vi "onDestroy.vi"(8 "error in (no error)":errorcluster, 11 "MeasuringDevice":refnum<class "MeasuringDevice.lvclass">) -> (0 "error out":errorcluster, 3 "MeasuringDevice out":refnum<class "MeasuringDevice.lvclass">)   [LabVIEW 2019, in "MeasuringDevice.lvclass"]
doc: "JKI State Machine Objects (SMO) 1.3.0.56\nJKI - JKI\nCopyright (c) 2017, JKI"
uses:
  MeasuringDevice.lvclass
  CircularBuffer/CircularBuffer.lvclass
  C:/Program Files (x86)/National Instruments/LabVIEW 2019/vi.lib/JKI/JKI SMO/SMO/SMO.lvclass
  Device/Device.lvclass
  <vilib>/JKI/JKI SMO/SMO/SMO.lvclass
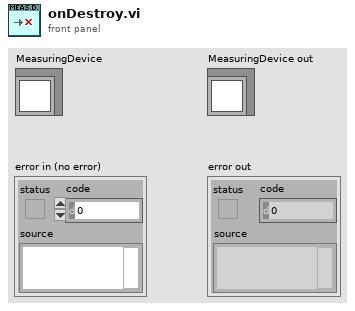
[diagram p1: front panel]
types:
  T1 = typedef "MeasuringDevice.lvclass/Dependencies--Cluster.ctl" = cluster{"MeasurementBuffer":refnum<class "CircularBuffer.lvclass">}
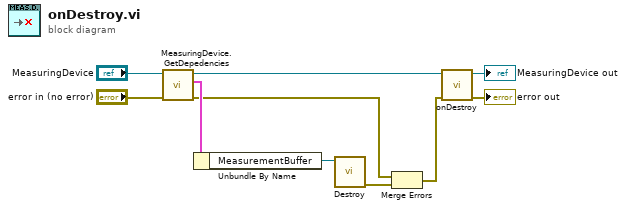
[diagram p0: block diagram]
diagram:
  n1 = call "MeasuringDevice.GetDepedencies.vi"("error in (no error)"="error in (no error)", "MeasuringDevice"="MeasuringDevice") -> ("error out"=w2:errorcluster, "Dependencies"=w5:T1, "MeasuringDevice"=w7:refnum<class "MeasuringDevice.lvclass">)  [unwired: 7 in]
  n2 = Unbundle By Name(w5) -> ("MeasurementBuffer"=w4:refnum<class "CircularBuffer.lvclass">)
  n3 = call <vilib>:"Destroy.vi"("SMO"=w4) -> ("error out"=w3:errorcluster)  [unwired: 10 in]
  n4 = Merge Errors(w2, w3) -> (w1:errorcluster)
  n5 = call-parent "onDestroy.vi"("error in (no error)"=w1, "SMO"=w7) -> ("error out"=→"error out":errorcluster, "SMO out"=→"MeasuringDevice out":refnum<class "MeasuringDevice.lvclass">)  [unwired: 8 in]
